vi "Visit_Shortcut.vi"(8 "error in (no error)":errorcluster, 10 "shortcut address":T1, 11 "Installer in":refnum<class "Installer.lvclass">) -> (0 "error out":errorcluster, 1 "file out":refnum<class "IB_Source_File.lvclass">, 2 "shortcut":refnum<class "IB_Shortcut.lvclass">, 3 "Installer out":refnum<class "Installer.lvclass">)   [LabVIEW 2020, in "Installer.lvclass"]
uses:
  <vilib>/AppBuilder/IB_Classes/Installer/Installer.lvclass
  <vilib>/AppBuilder/IB_Classes/Installer/Installer.lvclass/Installer.ctl
  <vilib>/AppBuilder/IB_Classes/Source/File/IB_Source_File.lvclass
  <vilib>/AppBuilder/IB_Classes/Shortcut/IB_Shortcut.lvclass
  <resource>/Framework/Providers/Builds/Installer/CDK_sTypeDef_ShortcutAddress.ctl
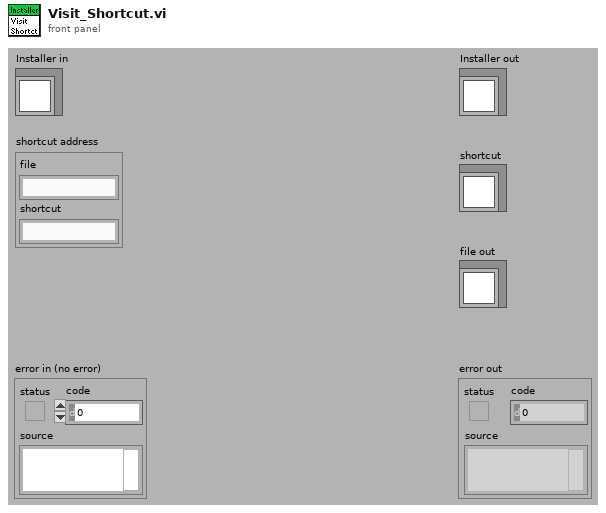
[diagram p1: front panel]
types:
  T1 = typedef "CDK_sTypeDef_ShortcutAddress.ctl" = cluster{"file":string, "shortcut":string}
  T2 = typedef "IB_Source_File.ctl" = cluster{"Attributes":i16, "RegCOM":bool, "unlock":bool, "shortcuts":refnum<class "IB_Shortcut.lvclass">[], "EXE_install":bool, "CmdArg_install":string, "EXE_uninstall":bool, "CmdArg_uninstall":string}
  T3 = typedef "IB_Shortcut.ctl" = cluster{"name":string, "destIndex":i32, "subDir":string, "address":string}
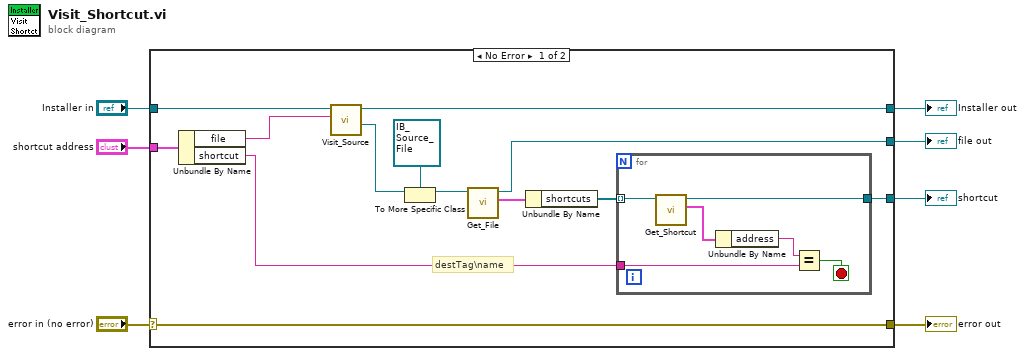
[diagram p0: block diagram]
diagram:
  n1 = case shown="No Error" "error in (no error)" {
    selector: "error in (no error)" -> [w20 w28]
    tunnel: [w20 w28] -> w6
    tunnel: [w18 w27] -> w4
    tunnel: "Installer in" -> [w19 w27]
    tunnel: "shortcut address" -> [w12 _]
    tunnel: [w13 _] -> w2
    tunnel: [w10 _] -> w1
    frame No Error {
      # "destTag\\name"
      n2 = Unbundle By Name(w12) -> ("file"=w9:string, "shortcut"=w11:string)
      n3 = call <vilib>:"Visit_Source.vi"("address"=w9, "Installer in"=w19) -> ("source"=w8:refnum<class "IB_Source.lvclass">, "Installer out"=w18:refnum<class "Installer.lvclass">)  [unwired: 1 in, 7 out]
      n4 = To More Specific Class(target class=refnum<class "IB_Source_File.lvclass"> refnum ("IB_Source_File.lvclass"), reference=w8) -> (specific class reference=w16:refnum<class "IB_Source_File.lvclass">)  [unwired: 1 in, 1 out]
      n5 = call <vilib>:"Get_File.vi"("IB_Source_File in"=w16) -> ("data"=w15:T2, "IB_Source_File out"=w10:refnum<class "IB_Source_File.lvclass">)  [unwired: 1 in, 8 out]
      n6 = Unbundle By Name(w15) -> ("shortcuts"=w14:refnum<class "IB_Shortcut.lvclass">[])
      n7 = for {
        tunnel: w14 -> [w26] mode=indexing
        tunnel: w11 -> [w24]
        tunnel: [w23] -> w13
        stop <- w22 stop-if-true
        n8 = call <vilib>:"Get_Shortcut.vi"("Class in"=w26) -> ("data"=w25:T3, "Class out"=w23:refnum<class "IB_Shortcut.lvclass">)  [unwired: 1 in, 8 out]
        n9 = Unbundle By Name(w25) -> ("address"=w21:string)
        n10 = Equal?(x=w21, y=w24) -> (x = y?=w22:bool)
      }
    }
    frame Error {
    }
  }
  "error out" <- w6
  "Installer out" <- w4
  "shortcut" <- w2
  "file out" <- w1
